vi "PH_Cam_BaseClass.update Cam Settings.vi"(0 "VI in":refnum<vi>, 2 "Cam Settings In":T1={"Cam ID"="N/A", "Gain"=nan, "Brightness"=nan, "Shutter"=nan, "Mode"=-1}, 5 "error in (no error)":errorcluster) -> (14 "VI out":refnum<vi>, 19 "error out":errorcluster)   [LabVIEW 2014, in "PH_Cam_BaseClass.lvlib"]
uses:
  PH_Cam_BaseClass.lvlib
  PH_Cam_BaseClass.Settings.ctl
  CSlibraries-extern/DimLVEvent/LVDimInterface/LVDimInterface.lvlib
  CS_Core/CSSystem/CoreLib/CoreLib.lvlib
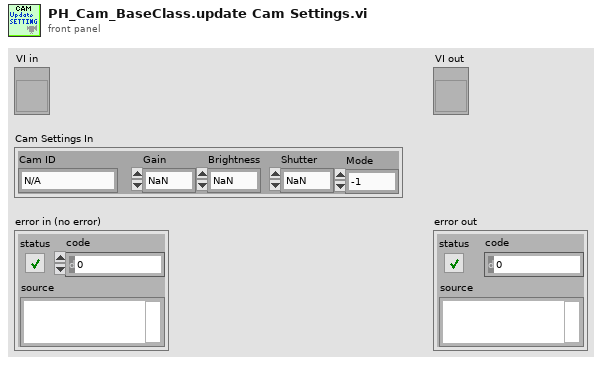
[diagram p1: front panel]
types:
  T1 = typedef "PH_Cam_BaseClass.lvlib/PH_Cam_BaseClass.Settings.ctl" = cluster{"Cam ID":string, "Gain":dbl, "Brightness":dbl, "Shutter":dbl, "Mode":i32}
  T2 = typedef "PH_Cam_BaseClass.lvlib/PH_Cam_BaseClass.i attribute.ctl" = cluster{"Gui Refs":T3, "Cam":cluster{"Source Notifier":refnum<notifier>, "Error":errorcluster, "Camera ID":string}, "Images":cluster{"Cam":T4, "Operation":T4, "PSDB":T4}, "Window Image":cluster{"Indicate Image":bool, "Window No.":i32, "Scale Facor":dbl, "Center Cross":bool, "Subtract Backgr":bool, "CoG":bool, "Color Palette":cluster{"Red":u8, "Green":u8, "Blue":u8}[], "Image On":bool}, "Default Prdc Int":i32, "Performance":cluster{"on":bool, "Timestamp Last Frame":i32}, "Histogram":cluster{"on":bool, "Mapping":bool}, "Save Image":cluster{"Save":bool, "File refnum":refnum<file>}, "Setting Service ID":i32, "Screen":cluster{"x-resolution":i16, "y-resolution":i16}, "On":bool, "Constructor finished":bool, "configured":bool}
  T3 = typedef "PH_Cam_BaseClass.lvlib/PH_Cam_BaseClass.GUI Refs.ctl" = cluster{"Frame Rate":refnum<vi>, "Get Frame Rate":refnum<vi>, "Show Image":refnum<vi>, "Get Histogram":refnum<vi>, "Mapping":refnum<vi>, "Histogram":refnum<vi>, "Center Cross":refnum<vi>, "Center of Gravity":refnum<vi>, "Scale Factor [%]":refnum<vi>, "Save Image":refnum<vi>, "Palette":refnum<vi>, "Subtract Background":refnum<vi>, "Cam Error":refnum<vi>, "On":refnum<vi>, "Cam List":refnum<vi>}
  T4 = typedef "IMAQ Image.ctl" = refnum<image>
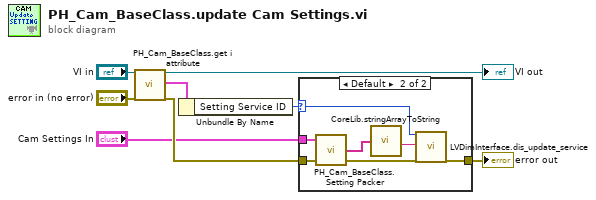
[diagram p0: block diagram]
diagram:
  n1 = call "PH_Cam_BaseClass.get i attribute.vi"("i ref in"="VI in", "error in (no error)"="error in (no error)") -> ("i ref out"=→"VI out":refnum<vi>, "i attribute"=w6:T2, "error out"=w5:errorcluster)  [unwired: 15 in]
  n2 = Unbundle By Name(w6) -> ("Setting Service ID"=w1:i32)
  n3 = case shown="Default" w1 {
    selector: w1 -> [_ w10]
    tunnel: [w9 w16] -> w8
    tunnel: w5 -> [w9 w13]
    tunnel: "Cam Settings In" -> [_ w11]
    frame -1 {
    }
    frame Default {
      n4 = call "PH_Cam_BaseClass.Setting Packer.vi"("error in (no error)"=w13, "Cam Settings In"=w11) -> ("error out"=w14:errorcluster, "Cam Settings"=w12:string[])  [unwired: 1 in, 1 out]
      n5 = call "CoreLib.stringArrayToString.vi"("Array"=w12) -> ("String"=w15:string)
      n6 = call "LVDimInterface.dis_update_service.vi"("my_serviceID"=w10, "data"=w15, "error in (no error)"=w14) -> ("error out"=w16:errorcluster)  [unwired: 14 in, 2 out]
    }
  }
  "error out" <- w8
